vi "SwerveDriveCalculations.vi"(11 "SwerveCommands":dbl[](array[numeric])) -> (1 "Velocity":dbl[](array[numeric]), 3 "Angle":dbl[](array[numeric]))   [LabVIEW 2020]
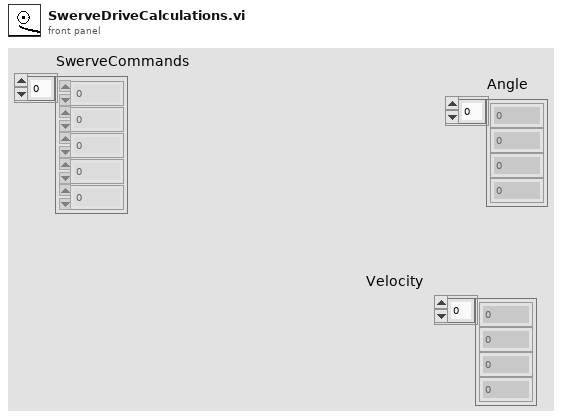
[diagram p1: front panel]
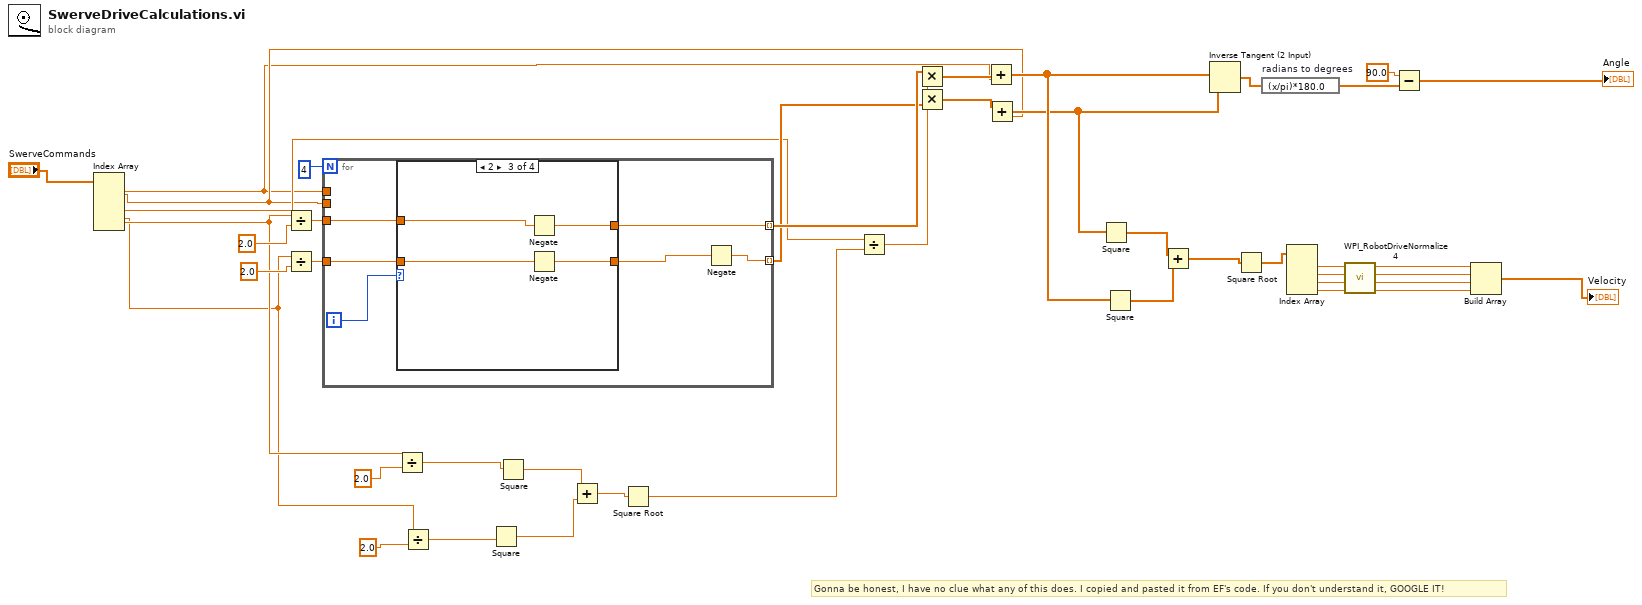
[diagram p0: block diagram]
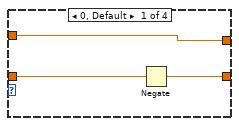
[diagram p2: hidden frame]
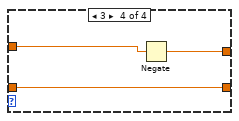
[diagram p4: hidden frame]
diagram:
  # "Gonna be honest, I have no clue what any of this does. I copied and pasted it from EF's code. If you don't understand it, GOOGLE IT!"
  n1 = Index Array(array="SwerveCommands") -> (element #1=w7:dbl, element #2=w6:dbl, element #3=w20:dbl, element #4=w4:dbl, element #5=w5:dbl)  [unwired: 5 in]
  n2 = Divide(x=w5, y=2.0) -> (x/y=w35:dbl)
  n3 = Divide(x=w4, y=2.0) -> (x/y=w34:dbl)
  n4 = for {
    N: 4 -> [_]
    tunnel: w35 -> [w47]
    tunnel: w34 -> [w46]
    tunnel: w6 -> [_]
    tunnel: w7 -> [_]
    tunnel: [w44] -> w24 mode=indexing
    tunnel: [w43] -> w25 mode=indexing
    i -> [w48]
    n5 = case shown="2" w48 {
      tunnel: w47 -> [w49 w52 w57 w60]
      tunnel: w46 -> [w51 w53 w55 w58]
      tunnel: [w50 w53 w54 w58] -> w45
      tunnel: [w49 w52 w56 w59] -> w43
      frame 0, Default {
        n6 = Negate(x=w51) -> (-x=w50:dbl)
      }
      frame 1 {
      }
      frame 2 {
        n7 = Negate(x=w57) -> (-x=w56:dbl)
        n8 = Negate(x=w55) -> (-x=w54:dbl)
      }
      frame 3 {
        n9 = Negate(x=w60) -> (-x=w59:dbl)
      }
    }
    n10 = Negate(x=w45) -> (-x=w44:dbl)
  }
  n11 = Divide(x=w5, y=2.0) -> (x/y=w30:dbl)
  n12 = Divide(x=w4, y=2.0) -> (x/y=w31:dbl)
  n13 = Square(x=w31) -> (x^2=w28:dbl)
  n14 = Square(x=w30) -> (x^2=w29:dbl)
  n15 = Add(x=w29, y=w28) -> (x+y=w27:dbl)
  n16 = Square Root(x=w27) -> (sqrt(x)=w8:dbl)
  n17 = Divide(x=w20, y=w8) -> (x/y=w26:dbl)
  n18 = Multiply(x=w25, y=w26) -> (x*y=w19:dbl[])
  n19 = Multiply(x=w26, y=w24) -> (x*y=w18:dbl[])
  n20 = Add(x=w19, y=w6) -> (x+y=w17:dbl[])
  n21 = Add(x=w18, y=w7) -> (x+y=w16:dbl[])
  n22 = Square(x=w16) -> (x^2=w15:dbl[])
  n23 = Square(x=w17) -> (x^2=w14:dbl[])
  n24 = Add(x=w15, y=w14) -> (x+y=w13:dbl[])
  n25 = Inverse Tangent (2 Input)(1:w16, 2:w17) -> (0:w22:dbl[])
  n26 = Square Root(x=w13) -> (sqrt(x)=w12:dbl[])
  n27 = expression code="(x/pi)*180.0" "radians to degrees"(w22) -> (w21:dbl[])
  n28 = Index Array(array=w12) -> (element #1=w11:dbl, element #3=w9:dbl, element #4=w10:dbl)  [unwired: 4 in, 1 out]
  n29 = call <vilib>:"WPI_RobotDriveNormalize 4.vi"("D"=w10, "C"=w9, "B"=w11, "A"=w11) -> ("D'"=w42:dbl, "C'"=w41:dbl, "B'"=w40:dbl, "A'"=w39:dbl)
  n30 = Subtract(x=90.0, y=w21) -> (x-y=→"Angle":dbl[])
  n31 = Build Array(w39, w40, w41, w42) -> (→"Velocity":dbl[])
